vi "AddData2StatArray.vi"(0 "Data2Process":string[][](array[string]), 7 "StatArrayIn":string[][](array[string])) -> (8 "StatArrayOut":string[][](array[string]))   [LabVIEW 2013]
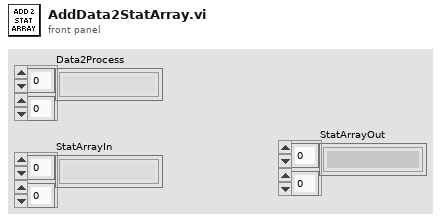
[diagram p1: front panel]
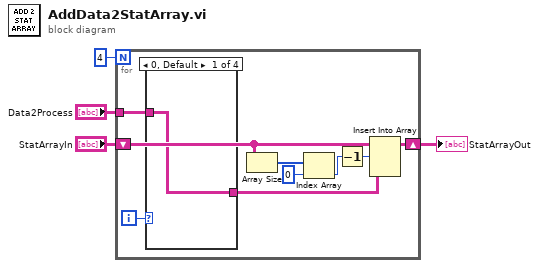
[diagram p0: block diagram]
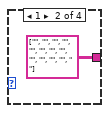
[diagram p2: hidden frame]
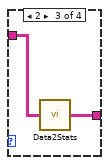
[diagram p3: hidden frame]
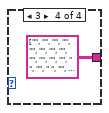
[diagram p4: hidden frame]
diagram:
  n1 = for {
    N: 4 -> [_]
    shift-right: [w12] -> w2
    shift-left: "StatArrayIn" -> [w8]
    tunnel: "Data2Process" -> [w7]
    i -> [w13]
    n2 = case shown="0, Default" w13 {
      tunnel: [w14 string[][] [["", "", "", "", "", "", "", "", "", "", "", "", " "]] w16 string[][] [["", "", "", "", "", "", "", "", "", "", "", "", " "], ["", " ", "", "", "", "", "", "", "", "", "", "", ""]]] -> w9
      tunnel: w7 -> [w14 _ w17 _]
      frame 0, Default {
      }
      frame 1 {
      }
      frame 2 {
        n3 = call "Data2Stats.vi"("DataIn"=w17) -> ("StatsOut"=w16:string[][])  [unwired: 14 in]
      }
      frame 3 {
      }
    }
    n4 = Array Size(array=w8) -> (size(s)=w11:i32[])
    n5 = Index Array(array=w11, index=0) -> (element=w6:i32)
    n6 = Decrement(x=w6) -> (x-1=w5:i32)
    n7 = Insert Into Array(array=w8, index (row)=w5, new element=w9) -> (w12:string[][])  [unwired: 1 in]
  }
  "StatArrayOut" <- w2
